vi "new_show_intern.vi"(7 "reference":refnum<vi>, 8 "lines":i32, 9 "x":i32, 10 "first letter to find":string="i", 11 "Array":string[](array[string])=["F", "a", "b", "i", "o"]) -> ()   [LabVIEW 2014]
uses:
  <vilib>/Utility/miscctls.llb/LVRowAndColumnUnsignedTypeDef.ctl
  <vilib>/Utility/miscctls.llb/LVRowAndColumnTypeDef.ctl
  <vilib>/Utility/miscctls.llb/LVBoundsTypeDef.ctl
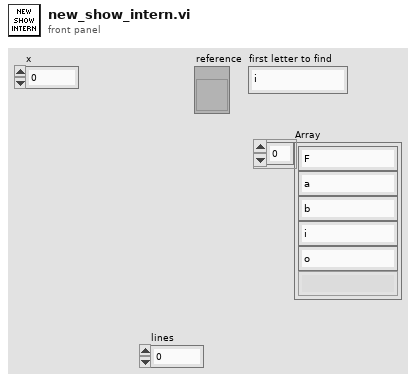
[diagram p1: front panel]
types:
  T1 = typedef "LVRowAndColumnUnsignedTypeDef.ctl" = cluster{"Row":u32, "Column":u32}
  T2 = typedef "LVBoundsTypeDef.ctl" = cluster{"Width":u32, "Height":u32}
  T3 = typedef "LVRowAndColumnTypeDef.ctl" = cluster{"Row":i32, "Column":i32}
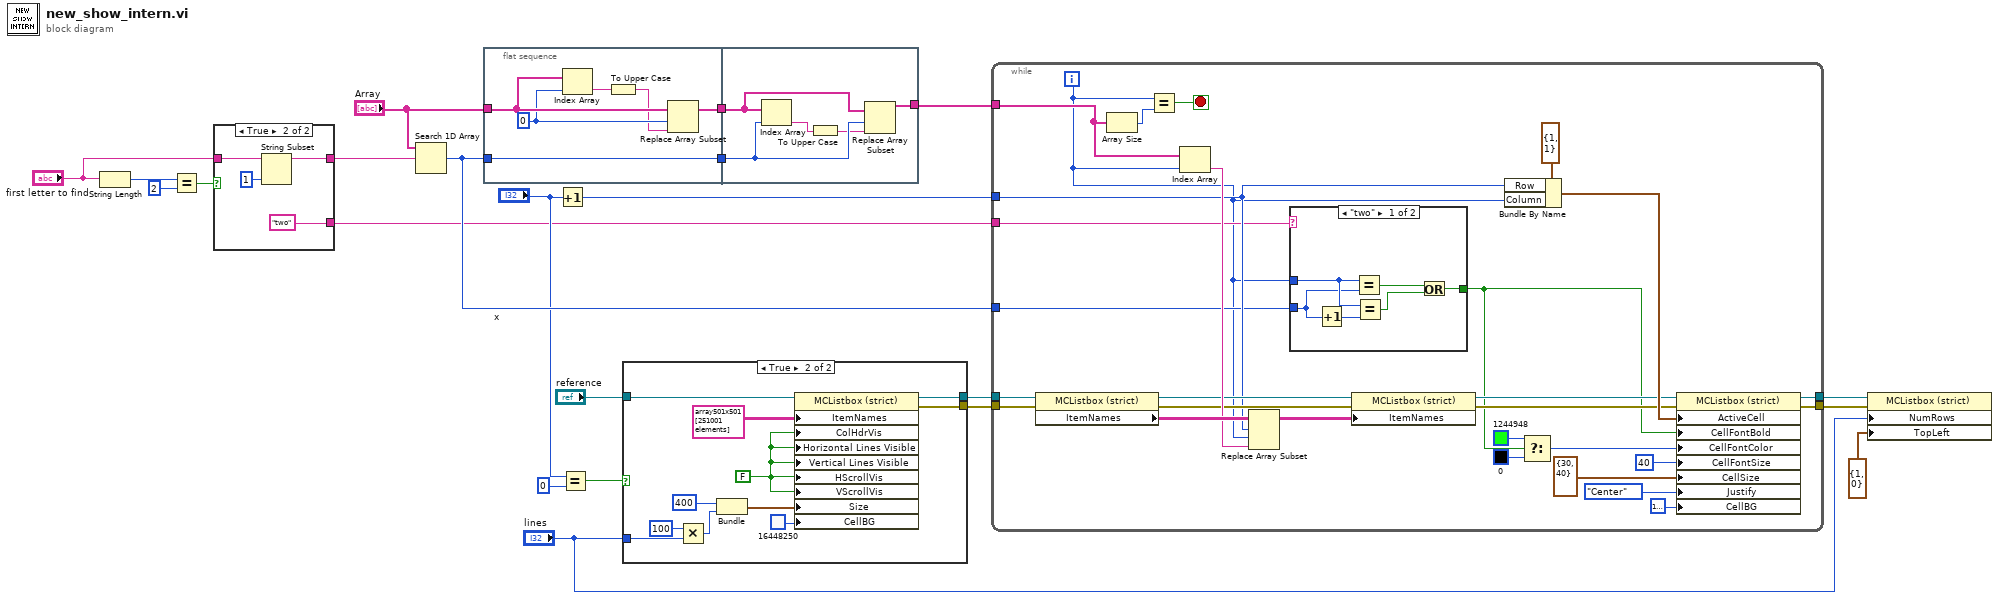
[diagram p0: block diagram]
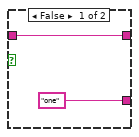
[diagram p2: hidden frame]
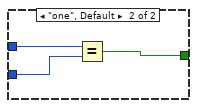
[diagram p4: hidden frame]
diagram:
  n1 = String Length(string="first letter to find") -> (length=w11:i32)
  n2 = Equal?(x=w11, y=2) -> (x = y?=w9:bool)
  n3 = case shown="True" w9 {
    tunnel: "first letter to find" -> [w24 w28]
    tunnel: [w24 w26] -> w7
    tunnel: ["one" "two"] -> w1
    frame False {
    }
    frame True {
      n4 = String Subset(string=w28, length (rest)=1 ("length (rest)")) -> (substring=w26:string)  [unwired: 1 in]
    }
  }
  n5 = Search 1D Array(1D array="Array", element=w7) -> (index of element=w17:i32)  [unwired: 1 in]
  n6 = flat-sequence {
    tunnel: "Array" -> [w34]
    tunnel: [w29] -> w22
    tunnel: [w30] -> w21
    tunnel: w17 -> [w30]
    tunnel: w22 -> [w39]
    tunnel: w21 -> [w38]
    tunnel: [w35] -> w15
    frame #0 {
      w33 = 0 ("index")
      n7 = Index Array(array=w34, index=w33) -> (element=w32:string)
      n8 = To Upper Case(1:w32) -> (0:w31:string)
      n9 = Replace Array Subset(array=w34, new element=w31, index=w33) -> (w29:string[])
    }
    frame #1 {
      n10 = Index Array(array=w39, index=w38) -> (element=w37:string)
      n11 = To Upper Case(1:w37) -> (0:w36:string)
      n12 = Replace Array Subset(array=w39, new element=w36, index=w38) -> (w35:string[])
    }
  }
  n13 = Increment(x="x") -> (x+1=w6:i32)
  n14 = Equal?(x="x", y=0) -> (x = y?=w14:bool)
  n15 = case shown="True" w14 {
    tunnel: [_ w50] -> w20
    tunnel: "reference" -> [w40 w49]
    tunnel: [w40 w48] -> w18
    tunnel: "lines" -> [_ w46]
    frame False {
    }
    frame True {
      w41 = FALSE
      n16 = Multiply(x=100, y=w46) -> (x*y=w44:i32)
      n17 = Bundle(400, w44) -> (w42:cluster{i32, i32})  [unwired: 1 in]
      n18 = property on="Property Node" class="MCListbox (strict)"(reference=w49, "ItemNames"=string[][] array501x501[251001 elements], "ColHdrVis"=w41, "Horizontal Lines Visible"=w41, "Vertical Lines Visible"=w41, "HScrollVis"=w41, "VScrollVis"=w41, "Size"=w42, "CellBG"=u32 16448250) -> (reference out=w48:refnum<vi>, error out=w50:errorcluster)  [unwired: 1 in]
    }
  }
  n19 = while {
    tunnel: w15 -> [w71]
    tunnel: w20 -> [w67]
    tunnel: w17 -> [w56]
    tunnel: [w68] -> w4
    tunnel: w18 -> [w58]
    tunnel: w6 -> [w57]
    tunnel: w1 -> [w55]
    tunnel: [w52] -> w3
    i -> [w53]
    stop <- w69 stop-if-true
    n20 = property on="Property Node" class="MCListbox (strict)"(reference=w58, error in=w67) -> (reference out=w59:refnum<vi>, error out=w66:errorcluster, "ItemNames"=w79:string[][])
    n21 = Array Size(array=w71) -> (size(s)=w70:i32)
    n22 = Equal?(x=w53, y=w70) -> (x = y?=w69:bool)
    n23 = Index Array(array=w71, index=w53) -> (element=w78:string)
    n24 = Replace Array Subset(array=w79, new element=w78, index (row)=w57, index (col)=w53) -> (w77:string[][])
    n25 = case shown="\"two\"" w55 {
      tunnel: w56 -> [w81 w88]
      tunnel: w53 -> [w83 w87]
      tunnel: [w80 w86] -> w54
      frame "two" {
        n26 = Increment(x=w81) -> (x+1=w82:i32)
        n27 = Equal?(x=w83, y=w81) -> (x = y?=w85:bool)
        n28 = Equal?(x=w83, y=w82) -> (x = y?=w84:bool)
        n29 = Or(x=w85, y=w84) -> (x .or. y?=w80:bool)
      }
      frame "one", Default {
        n30 = Equal?(x=w87, y=w88) -> (x = y?=w86:bool)
      }
    }
    n31 = property on="Property Node" class="MCListbox (strict)"(reference=w59, error in=w66, "ItemNames"=w77) -> (reference out=w60:refnum<vi>, error out=w65:errorcluster)
    n32 = Bundle By Name(cluster=T3 {"Row"=1, "Column"=1} ("Active Cell:Active Cell"), "Row"=w57, "Column"=w53) -> (w75:T3)
    n33 = Select(t=u32 1244948, s=w54, f=u32 0) -> (s? t:f=w63:u32)
    n34 = property on="Property Node" class="MCListbox (strict)"(reference=w60, error in=w65, "ActiveCell"=w75, "CellFontBold"=w54, "CellFontColor"=w63, "CellFontSize"=u32 40 ("Active Cell:Cell Font:Size"), "CellSize"=T2 {"Width"=30, "Height"=40} ("Active Cell:Cell Size"), "Justify"=enum16{"Left", "Center", "Right"}."Center" ("Active Cell:Cell Justification"), "CellBG"=u32 16777226) -> (reference out=w52:refnum<vi>, error out=w68:errorcluster)
  }
  n35 = property on="Property Node" class="MCListbox (strict)"(reference=w3, error in=w4, "NumRows"="lines", "TopLeft"=T1 {"Row"=1, "Column"=0} ("Top Left Visible Cell")) -> ()  [unwired: 2 out]
